vi "Get LabVIEW versions.vi"(8 "error in (no error)":errorcluster) -> (0 "error out":errorcluster, 3 "LV Version Details":T1[](array[typedef]))   [LabVIEW 2016]
uses:
  TypeDefs/LV Version Details.ctl
  <vilib>/registry/registry.llb/Registry View.ctl
  <vilib>/registry/registry.llb/Registry RtKey.ctl
  <vilib>/registry/registry.llb/Registry SAM.ctl
  <vilib>/registry/registry.llb/Read Registry Value Simple STR.vi
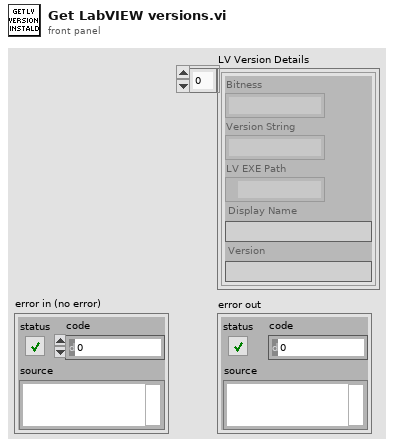
[diagram p1: front panel]
types:
  T1 = typedef "LV Version Details.ctl" = cluster{"Bitness":string, "Version String":string, "LV EXE Path":path, "Display Name":string, "Version":string}
  T2 = typedef "Registry View.ctl" = u16
  T3 = typedef "Registry SAM.ctl" = enum32{"KEY_QUERY_VALUE", "KEY_SET_VALUE", "KEY_CREATE_SUB_KEY", "KEY_ENUMERATE_SUB_KEYS", "KEY_NOTIFY", "KEY_CREATE_LINK", "KEY_READ", "KEY_WRITE", "KEY_ALL_ACCESS", "KEY_READ | KEY_WRITE"}
  T4 = typedef "Registry RtKey.ctl" = enum32{"HKEY_CLASSES_ROOT", "HKEY_CURRENT_USER", "HKEY_LOCAL_MACHINE", "HKEY_USERS", "HKEY_PERFORMANCE_DATA", "HKEY_CURRENT_CONFIG", "HKEY_DYN_DATA"}
  T5 = typedef "Registry refnum.ctl" = refnum<k1>
  T6 = cluster{"numSubKeys":i32, "maxSubKeyLen":i32, "maxSubKeyClassLen":i32}
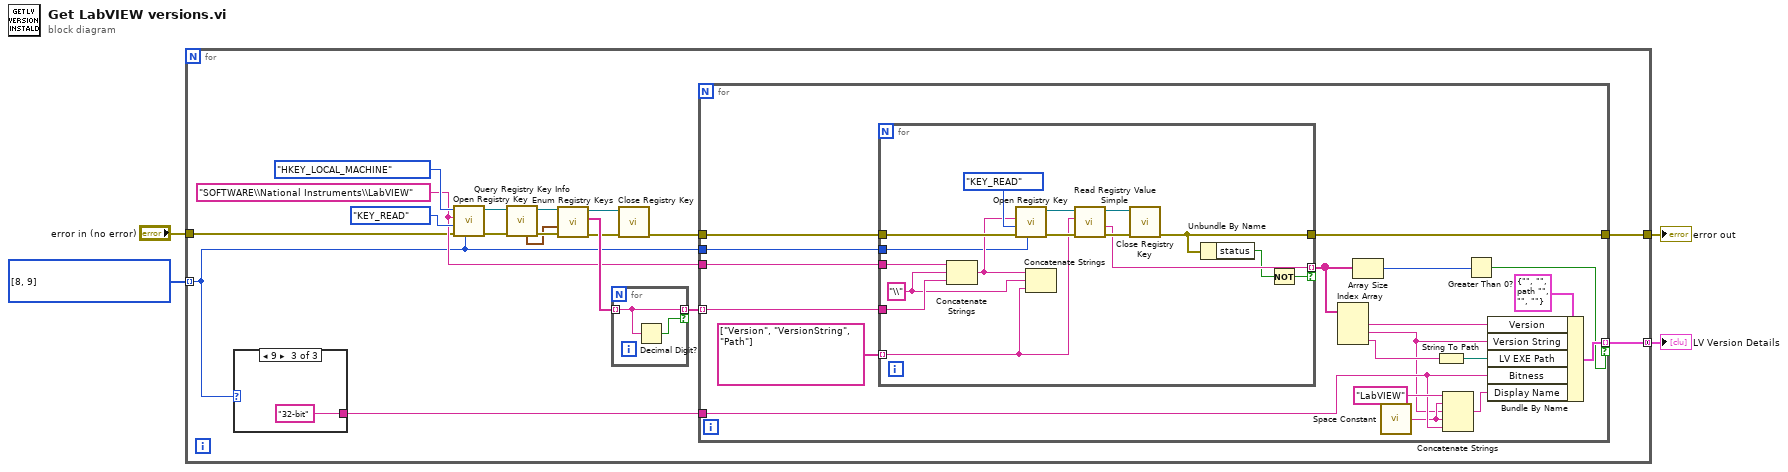
[diagram p0: block diagram]
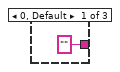
[diagram p2: hidden frame]
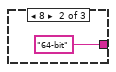
[diagram p3: hidden frame]
diagram:
  w4 = T2[] [8, 9] items=["Default"=0, "KEY_WOW64_64KEY"=8, "KEY_WOW64_32KEY"=9]
  n1 = for {
    tunnel: w4 -> [w7] mode=indexing
    tunnel: [w9] -> w3
    tunnel: "error in (no error)" -> [w8]
    tunnel: [w5] -> w1 mode=concatenating
    w10 = "SOFTWARE\\National Instruments\\LabVIEW" ("subkey")
    n2 = case shown="9" w7 {
      tunnel: ["" "64-bit" "32-bit"] -> w6
      frame 0, Default {
      }
      frame 8 {
      }
      frame 9 {
      }
    }
    n3 = call <vilib>:"Open Registry Key.vi"("registry view"=w7, "error in (no error)"=w8, "security access mask (KEY_READ | KEY_WRITE)"=Registry_SAM."KEY_READ", "subkey"=w10, "root key (HKEY_LOCAL_MACHINE)"=Registry_RtKey."HKEY_LOCAL_MACHINE") -> ("error out"=w22:errorcluster, "refnum out"=w21:T5)  [unwired: 5 in]
    n4 = call <vilib>:"Query Registry Key Info.vi"("error in (no error)"=w22, "refnum"=w21) -> ("error out"=w18:errorcluster, "refnum out"=w17:T5, "subkey info"=w16:T6)  [unwired: 5 in, 2 out]
    n5 = call <vilib>:"Enum Registry Keys.vi"("error in (no error)"=w18, "subkey info"=w16, "refnum"=w17) -> ("error out"=w14:errorcluster, "subkeys"=w15:string[], "refnum out"=w13:T5)  [unwired: 6 in]
    n6 = for {
      tunnel: w15 -> [w62] mode=indexing
      tunnel: [w62] -> w11 mode=indexing if=w61
      n7 = Decimal Digit?(1:w62) -> (0:w61:bool)
    }
    n8 = call <vilib>:"Close Registry Key.vi"("error in (no error)"=w14, "refnum"=w13) -> ("error out"=w12:errorcluster)  [unwired: 5 in]
    n9 = for {
      tunnel: w12 -> [w44]
      tunnel: w11 -> [w42] mode=indexing
      tunnel: w10 -> [w43]
      tunnel: [w40] -> w9
      tunnel: [w37] -> w5 mode=indexing if=w33
      tunnel: w7 -> [w36]
      tunnel: w6 -> [w31]
      n10 = for {
        tunnel: w44 -> [w60]
        tunnel: w43 -> [w59]
        tunnel: [w50] -> w35 mode=indexing if=w46
        tunnel: w42 -> [w57]
        tunnel: string[] ["Version", "VersionString", "Path"] -> [w49] mode=indexing
        tunnel: [w48] -> w40
        tunnel: w36 -> [w45]
        w51 = "\\" ("string")
        n11 = Concatenate Strings(w59, w51, w57) -> (w52:string)
        n12 = call <vilib>:"Open Registry Key.vi"("registry view"=w45, "error in (no error)"=w60, "security access mask (KEY_READ | KEY_WRITE)"=Registry_SAM."KEY_READ", "subkey"=w52) -> ("error out"=w56:errorcluster, "refnum out"=w55:T5)  [unwired: 6 in]
        n13 = Concatenate Strings(w52, w51, w49) -> ()  [unwired: 1 out]
        n14 = call-poly <vilib>:"Read Registry Value Simple.vi"("error in (no error)"=w56, "value"=w49, "refnum"=w55) -> ("error out"=w54:errorcluster, "String/Binary data"=w50:string, "refnum out"=w53:T5)  [unwired: 3 in, 1 out]
        n15 = call <vilib>:"Close Registry Key.vi"("error in (no error)"=w54, "refnum"=w53) -> ("error out"=w48:errorcluster)  [unwired: 5 in]
        n16 = Unbundle By Name(w48) -> ("status"=w47:bool)
        n17 = Not(x=w47) -> (.not. x?=w46:bool)
      }
      n18 = Index Array(array=w35) -> (element #1=w26:string, element #2=w27:string, element #3=w28:string)  [unwired: 3 in]
      n19 = Array Size(array=w35) -> (size(s)=w34:i32)
      n20 = call <vilib>:"Space Constant.vi"() -> ("String"=w30:string)
      n21 = String To Path(string=w28) -> (path=w38:path)
      n22 = Concatenate Strings("LabVIEW" ("string"), w30, w27, w30, w31) -> (w29:string)
      n23 = Greater Than 0?(x=w34) -> (x > 0?=w33:bool)
      n24 = Bundle By Name(cluster=T1 {"Bitness"="", "Version String"="", "LV EXE Path"=path "", "Display Name"="", "Version"=""}, "Version"=w26, "Version String"=w27, "LV EXE Path"=w38, "Bitness"=w31, "Display Name"=w29) -> (w37:T1)
    }
  }
  "error out" <- w3
  "LV Version Details" <- w1
